vi "New Heading 3 Object.vi"(8 "error in (no error)":errorcluster) -> (0 "error out":errorcluster, 3 "Heading 3 out":refnum<class "Heading 3.lvclass">)   [LabVIEW 2017, in "Styles.lvlib" / "Heading 3.lvclass"]
uses:
  Heading 3.lvclass
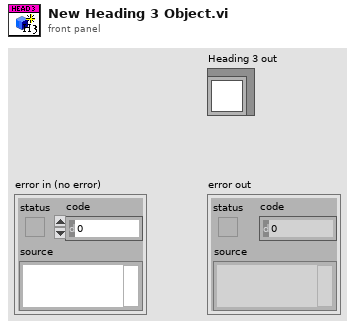
[diagram p1: front panel]
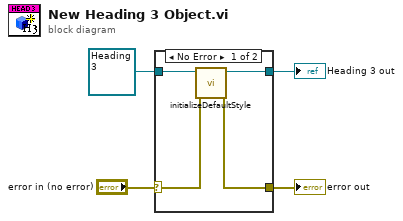
[diagram p0: block diagram]
diagram:
  n1 = case shown="No Error" "error in (no error)" {
    selector: "error in (no error)" -> [w7 w10]
    tunnel: refnum<class "Heading 3.lvclass"> refnum ("Heading 3 in") -> [w8 w9]
    tunnel: [w6 w10] -> w1
    tunnel: [w5 w9] -> w3
    frame No Error {
      n2 = call-dynamic "initializeDefaultStyle.vi"("error in (no error)"=w7, "Heading 3 in"=w8) -> ("error out"=w6:errorcluster, "Heading 3 out"=w5:refnum<class "Heading 3.lvclass">)  [unwired: 8 in]
    }
    frame Error {
    }
  }
  "error out" <- w1
  "Heading 3 out" <- w3
